vi "Hailo_main_calib.vi"(10 "Sensor Readings (Signed)":i16[](array[numeric])) -> (2 "Sensor Readings":dbl[][](array[numeric])=[[-533.0, -111.0, 239.0], [-402.0, 166.0, 184.0], [-184.0, 154.0, 29.0], [-106.0, 74.0, 11.0], [-532.0, -109.0, 246.0], [-398.0, 164.0, 175.0], [-205.0, 152.0, 32.0], [-119.0, 65.0, 9.0], [-529.0, -110.0, 242.0], [-408.0, 166.0, 184.0], [-198.0, 158.0, 27.0], [-108.0, 61.0, 6.0], [-539.0, -106.0, 240.0], [-407.0, 158.0, 183.0], [-191.0, 156.0, 28.0], [-113.0, 73.0, 15.0], [816.0, -260.0, 842.0], [539.0, 512.0, 512.0], [156.0, 425.0, 83.0], [13.0, 142.0, -72.0], [816.0, -262.0, 840.0], [528.0, 520.0, 512.0], [162.0, 425.0, 83.0], [13.0, 137.0, -84.0], [809.0, -260.0, 840.0], [538.0, 520.0, 504.0], [162.0, 432.0, 72.0], [13.0, 136.0, -84.0], [809.0, -260.0, 846.0], [538.0, 508.0, 512.0], [158.0, 435.0, 72.0], [19.0, 136.0, -79.0], [346.0, -168.0, 14.0], [287.0, -68.0, 19.0], [161.0, -34.0, 4.0], [70.0, -44.0, -7.0], [345.0, -191.0, 19.0], [279.0, -40.0, 8.0], [167.0, -16.0, 12.0], [72.0, -23.0, 2.0], [341.0, -190.0, 17.0], [285.0, -46.0, 9.0], [149.0, -15.0, 6.0], [54.0, -40.0, -2.0], [375.0, -201.0, 19.0], [282.0, -51.0, 10.0], [135.0, -37.0, 6.0], [81.0, -57.0, -12.0], [-80.0, -193.0, -48.0], [-73.0, -136.0, -12.0], [-5.0, -122.0, -31.0], [-19.0, -118.0, -17.0], [-118.0, -187.0, -48.0], [-73.0, -115.0, -22.0], [1.0, -113.0, -27.0], [-20.0, -111.0, -8.0], [-99.0, -184.0, -40.0], [-62.0, -145.0, -17.0], [0.0, -113.0, -37.0], [-7.0, -117.0, -15.0], [-126.0, -184.0, -50.0], [-72.0, -115.0, -14.0], [-4.0, -114.0, -25.0], [-29.0, -116.0, -14.0]])   [LabVIEW 2016]
uses:
  FGVs/FGV States.ctl
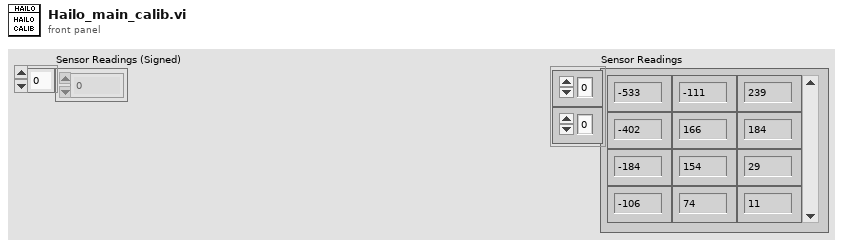
[diagram p1: front panel]
types:
  T1 = typedef "FGV States.ctl" = enum16{"Get", "Set", "Reset"}
  T2 = cluster{cluster{dbl[][], "Array":dbl[][]}, cluster{dbl[][], "Array":dbl[][]}, cluster{dbl[][], "Array":dbl[][]}, cluster{dbl[][], "Array":dbl[][]}}[]
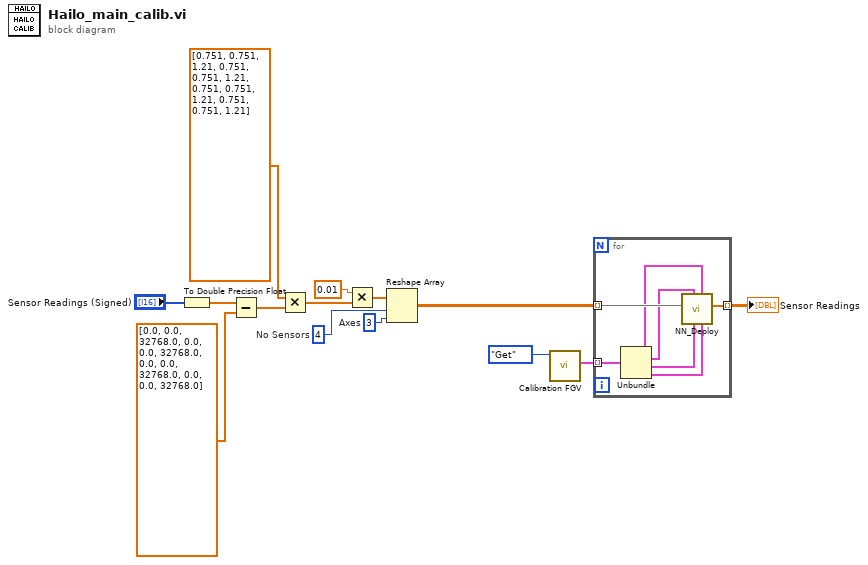
[diagram p0: block diagram]
diagram:
  w14 = 4  # No Sensors
  w13 = 3  # Axes
  n1 = To Double Precision Float(number="Sensor Readings (Signed)") -> (double precision float=w6:dbl[])
  n2 = Subtract(x=w6, y=dbl[] [0.0, 0.0, 32768.0, 0.0, 0.0, 32768.0, 0.0, 0.0, 32768.0, 0.0, 0.0, 32768.0]) -> (x-y=w8:dbl[])
  n3 = Multiply(x=dbl[] [0.751, 0.751, 1.21, 0.751, 0.751, 1.21, 0.751, 0.751, 1.21, 0.751, 0.751, 1.21], y=w8) -> (x*y=w3:dbl[])
  n4 = Multiply(x=0.01, y=w3) -> (x*y=w9:dbl[])
  n5 = Reshape Array(w9, w14, w13) -> (w12:dbl[][])
  n6 = call "Calibration FGV.vi"("FGV States"=FGV_States."Get") -> ("Calib in 2"=w4:T2)  [unwired: 10 in]
  n7 = for {
    tunnel: w12 -> [w21] mode=indexing
    tunnel: [w20] -> w10 mode=indexing
    tunnel: w4 -> [w19] mode=indexing
    n8 = Unbundle(w19) -> (w18:cluster{dbl[][], "Array":dbl[][]}, w17:cluster{dbl[][], "Array":dbl[][]}, w16:cluster{dbl[][], "Array":dbl[][]}, w15:cluster{dbl[][], "Array":dbl[][]})
    n9 = call "NN_Deploy.vi"("Output Layer"=w15, "Input Layer"=w18, "Layer 2"=w16, "Layer 1"=w17, "Input"=w21) -> ("Output"=w20:dbl[])  [unwired: 6 in]
  }
  "Sensor Readings" <- w10
